vi "Create Kernel Module LVLib.vi"(7 "Template LVLib Path":path=path "D:/Development/Projects/LQWidgets-CodeGen/templates/LabVIEW/Template.lvlib", 10 "Output Dir":path=path "D:/Development/Projects/LQWidgets/src/LabVIEW", 11 "Module Spec. File":path=path "D:/Development/Projects/LQWidgets-CodeGen/data/LQ Core.json") -> (1 "Manifestation Ancestors":T1, 2 "Module LVLib Path":path)   [LabVIEW 2013]
uses:
  Data Structures/Manifestation Ancestors.ctl
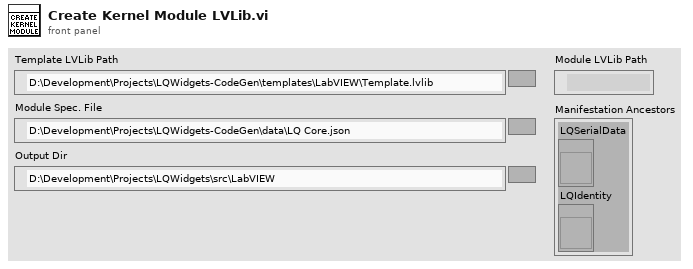
[diagram p1: front panel]
types:
  T1 = typedef "Manifestation Ancestors.ctl" = cluster{"LQSerialData":refnum<vi>, "LQIdentity":refnum<vi>}
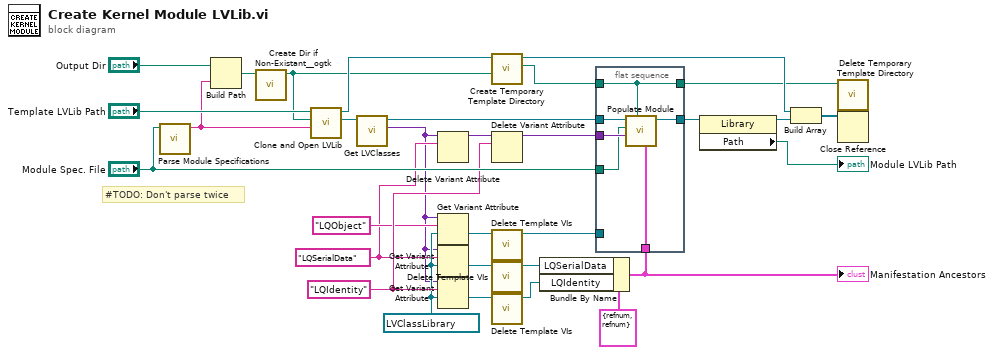
[diagram p0: block diagram]
diagram:
  w5 = refnum<vi> refnum ("Object Ref")
  w3 = "LQSerialData" ("name")
  w7 = "LQIdentity" ("name")
  # "#TODO: Don't parse twice"
  n1 = call "Parse Module Specifications.vi"("Module Spec. File"="Module Spec. File") -> ("Module Name"=w23:string)  [unwired: 7 in, 3 out]
  n2 = Build Path(base path="Output Dir", name or relative path=w23) -> (appended path=w22:path)
  n3 = call <userlib>:"Create Dir if Non-Existant__ogtk.vi"("Directory Path"=w22) -> ("dup Directory Path"=w16:path)  [unwired: 8 in, 2 out]
  n4 = call "Clone and Open LVLib.vi"("Output LVLib Name"=w23, "Output LVLib Dir"=w16, "Template LVLib Path"="Template LVLib Path") -> ("New LVLib"=w31:refnum<vi>, "Template LVLib"=w30:refnum<vi>)  [unwired: 7 in]
  n5 = call "Get LVClasses.vi"("LVLib"=w31) -> ("Class Ref Map"=w2:variant, "LVLib Dup"=w29:refnum<vi>)  [unwired: 9 in]
  n6 = Delete Variant Attribute(6:w3, 7:w2) -> (3:w9:variant)  [unwired: 1 in, 2 out]
  n7 = Get Variant Attribute(Variant=w2, name="LQObject", default value (empty Variant)=w5) -> (value=w4:refnum<vi>)  [unwired: 1 in, 3 out]
  n8 = Get Variant Attribute(Variant=w2, name=w3, default value (empty Variant)=w5) -> (value=w13:refnum<vi>)  [unwired: 1 in, 3 out]
  n9 = Get Variant Attribute(Variant=w2, name=w7, default value (empty Variant)=w5) -> (value=w11:refnum<vi>)  [unwired: 1 in, 3 out]
  n10 = call "Create Temporary Template Directory.vi"("Kernel LVLib Dir"=w16, "Template LVLib"=w30) -> ("Temporary Template Root Dir"=w26:path, "Template LVLib Dup"=w25:refnum<vi>)  [unwired: 8 in]
  n11 = Delete Variant Attribute(6:w7, 7:w9) -> (3:w8:variant)  [unwired: 1 in, 2 out]
  n12 = call "Delete Template VIs.vi"("LVClass"=w4) -> ("LVClass Dup"=w1:refnum<vi>)  [unwired: 10 in]
  n13 = call "Delete Template VIs.vi"("LVClass"=w13) -> ("LVClass Dup"=w12:refnum<vi>)  [unwired: 10 in]
  n14 = call "Delete Template VIs.vi"("LVClass"=w11) -> ("LVClass Dup"=w10:refnum<vi>)  [unwired: 10 in]
  n15 = Bundle By Name(cluster=T1 {"LQSerialData"=refnum, "LQIdentity"=refnum} ("Manifestation Ancestors"), "LQSerialData"=w12, "LQIdentity"=w10) -> (w14:T1)
  "Manifestation Ancestors" <- w14
  n16 = flat-sequence {
    tunnel: w29 -> [w37]
    tunnel: w8 -> [w36]
    tunnel: w26 -> [w33]
    tunnel: "Module Spec. File" -> [w35]
    tunnel: [w34] -> w20
    tunnel: [w33] -> w18
    tunnel: w14 -> [w32]
    tunnel: w1 -> [_]
    frame #0 {
      n17 = call "Populate Module.vi"("Manifestation Ancestors"=w32, "Temporary Template Root Dir"=w33, "Preloaded Module Class Ref Map"=w36, "Module Spec. File"=w35, "Module LVLib"=w37) -> ("Module LVLib Dup"=w34:refnum<vi>)  [unwired: 6 in]
    }
  }
  n18 = property class="Library"(reference=w20) -> (reference out=w19:refnum<vi>, "Path"=→"Module LVLib Path":path)  [unwired: 1 in, 1 out]
  n19 = Build Array(w25, w19) -> (w28:refnum<vi>[])
  n20 = call "Delete Temporary Template Directory.vi"("Target Template Root Dir"=w18) -> ()  [unwired: 11 in]
  n21 = Close Reference(reference=w28) -> ()  [unwired: 1 in, 1 out]
